vi "PathPlanner_Trajectory25_New.vi"(8 "RobotConfig":T1 {"moduleLocations"."Y" format="%14.3f"; "moduleLocations"."X" format="%14.3f"; "ModuleConfig"."driveMotor"."Jr_KgM2" format="%13.5p"; "ModuleConfig"."driveMotor"."L_H" format="%13.5p"; "ModuleConfig"."driveMotor"."Kt_NMPerAmp" format="%13.5p"; "ModuleConfig"."driveMotor"."KvINV_RadPerSecPerVolt" format="%13.5p"; "ModuleConfig"."driveMotor"."R_Ohms" format="%13.5p"; "ModuleConfig"."driveMotor"."FreeSpeed_RadPerSec" format="%13.5p"; "ModuleConfig"."driveMotor"."FreeCurrent_Amps" format="%13.5p"; "ModuleConfig"."driveMotor"."StallCurrent_Amps" format="%13.5p"; "ModuleConfig"."driveMotor"."StallTorque_NM" format="%13.5p"; "ModuleConfig"."driveMotor"."nominalVoltage_Volts" format="%13.5p"}, 9 "StartingRotation":T5={"VALUE"=0.0, "COS"=1.0, "SIN"=0.0} {"SIN" format="%13.4f"; "COS" format="%13.4f"; "VALUE" format="%13.4f"}, 10 "StartingSpeeds":T10 {"vOmega" format="%10.3f"; "vY" format="%10.3f"; "vX" format="%10.3f"}, 11 "Path":T11={"Reversed"=FALSE, "RotationTargets"=[], "ConstraintZones"=[], "EventMarkers"=[], "GlobalConstraints"={"MaxVelocityMps;"=0.0, "MaxAccelerationMpsSq;"=0.0, "MaxAngularVelRadPsEc;"=0.0, "MaxAngularAccRadPSecSq"=0.0, "Exists"=FALSE, "Unlimited"=FALSE, "NominalVoltageVolts"=12.0}, "GoalEndState"={"VelocityMPS"=0.0, "Rotation"={"VALUE"=0.0, "COS"=1.0, "SIN"=0.0}}, "AllPoints"=[], "Name"="", "Waypoints"=[], "PointTowardsZones"=[], "IdealStartingState"={"VelocityMPS"=0.0, "Rotation"={"VALUE"=1.0, "COS"=0.0, "SIN"=0.0}}, "IsChoreoPath"=FALSE, "PreventFlipping"=FALSE} {"IdealStartingState"."Rotation"."SIN" format="%13.4f"; "IdealStartingState"."Rotation"."COS" format="%13.4f"; "IdealStartingState"."Rotation"."VALUE" format="%13.4f"; "PointTowardsZones"."TargetPosition"."Y" format="%14.3f"; "PointTowardsZones"."TargetPosition"."X" format="%14.3f"; "PointTowardsZones"."RotationOffset"."SIN" format="%13.4f"; "PointTowardsZones"."RotationOffset"."COS" format="%13.4f"; "PointTowardsZones"."RotationOffset"."VALUE" format="%13.4f"; "Waypoints"."nextControl"."Y" format="%14.3f"; "Waypoints"."nextControl"."X" format="%14.3f"; "Waypoints"."anchor"."Y" format="%14.3f"; "Waypoints"."anchor"."X" format="%14.3f"; "Waypoints"."prevControl"."Y" format="%14.3f"; "Waypoints"."prevControl"."X" format="%14.3f"; "AllPoints"."RotationTarget"."rotation"."SIN" format="%13.4f"; "AllPoints"."RotationTarget"."rotation"."COS" format="%13.4f"; "AllPoints"."RotationTarget"."rotation"."VALUE" format="%13.4f"; "AllPoints"."Position"."Y" format="%14.3f"; "AllPoints"."Position"."X" format="%14.3f"; "GoalEndState"."Rotation"."SIN" format="%13.4f"; "GoalEndState"."Rotation"."COS" format="%13.4f"; "GoalEndState"."Rotation"."VALUE" format="%13.4f"; "RotationTargets"."rotation"."SIN" format="%13.4f"; "RotationTargets"."rotation"."COS" format="%13.4f"; "RotationTargets"."rotation"."VALUE" format="%13.4f"}) -> (1 "PathPlannerTrajectoryEvents":T6, 3 "PathPlannerTrajectory":T21 {"States"."ModuleStates"."SWERVE_DRIVE_MODULE_STATE"."Angle"."SIN" format="%13.4f"; "States"."ModuleStates"."SWERVE_DRIVE_MODULE_STATE"."Angle"."COS" format="%13.4f"; "States"."ModuleStates"."SWERVE_DRIVE_MODULE_STATE"."Angle"."VALUE" format="%13.4f"; "States"."ModuleStates"."FieldAngle"."SIN" format="%13.4f"; "States"."ModuleStates"."FieldAngle"."COS" format="%13.4f"; "States"."ModuleStates"."FieldAngle"."VALUE" format="%13.4f"; "States"."ModuleStates"."FieldPos"."Y" format="%14.3f"; "States"."ModuleStates"."FieldPos"."X" format="%14.3f"; "States"."DeltaRot"."SIN" format="%13.4f"; "States"."DeltaRot"."COS" format="%13.4f"; "States"."DeltaRot"."VALUE" format="%13.4f"; "States"."pose"."ROTATION"."SIN" format="%13.4f"; "States"."pose"."ROTATION"."COS" format="%13.4f"; "States"."pose"."ROTATION"."VALUE" format="%13.4f"; "States"."pose"."TRANSLATION"."Y" format="%14.3f"; "States"."pose"."TRANSLATION"."X" format="%14.3f"; "States"."FieldSpeeds"."vOmega" format="%10.3f"; "States"."FieldSpeeds"."vY" format="%10.3f"; "States"."FieldSpeeds"."vX" format="%10.3f"; "States"."Heading"."SIN" format="%13.4f"; "States"."Heading"."COS" format="%13.4f"; "States"."Heading"."VALUE" format="%13.4f"})   [LabVIEW 2019, in "PathPlanner24.lvlib"]
doc: "Generate a PathPlannerTrajectory\n\nInputs: \n - path - cluster - path to generate the trajectory for\n - startingSpeeds - chassis speeds - Starting speeds of the robot when starting the trajectory\n\nOutputs:\n - trajectory - cluster - created trajectory data\n - TrajectoryEvents - cluster - created trajectory events data cluster"
uses:
  PathPlanner24.lvlib
  <vilib>/Rock Robotics/WPI/ThirdParty/JAS_Junk/TrajLib/TypeDef/TRANSLATION2D.ctl
  <vilib>/Rock Robotics/WPI/ThirdParty/JAS_Junk/TrajLib/Trajectory_Library.lvlib
  <vilib>/Rock Robotics/WPI/ThirdParty/JAS_Junk/TrajLib/TypeDef/ROTATION2D.ctl
  TypeDef/PathPlannerPathConstraints.ctl
  ENum/PathPlanner_CommandUtilType_ENUM.ctl
  TypeDef/PathPlannerCommandUtil.ctl
  TypeDef/PathPlannerTrajectoryEvent.ctl
  TypeDef/PathPlannerTrajectoryEvents.ctl
  <vilib>/Rock Robotics/WPI/ThirdParty/JAS_Junk/TrajLib/TypeDef/CHASSIS_SPEEDS.ctl
  <vilib>/Rock Robotics/WPI/ThirdParty/JAS_Junk/TrajLib/TypeDef/POSE2D.ctl
  <vilib>/Rock Robotics/WPI/ThirdParty/JAS_Junk/TrajLib/TypeDef/SWERVE_DRIVE_MODULE_STATE.ctl
  TypeDef/PathPlannerSwerveModTrajState.ctl
  TypeDef/PathPlannerDriveFeedFwds.ctl
  TypeDef/PathPlannerTrajectoryState25.ctl
  TypeDef/PathPlannerTrajectory25.ctl
  TypeDef/PathPlannerRotationTarget.ctl
  TypeDef/PathPlannerConstraintsZone.ctl
  TypeDef/PathPlannerEventMarker.ctl
  TypeDef/PathPlannerGoalEndState.ctl
  TypeDef/PathPlannerPathPoint.ctl
  TypeDef/PathPlannerPath.ctl
  TypeDef/PathPlannerWaypoint.ctl
  TypeDef/PathPlannerPointTowardsZone.ctl
  TypeDef/PathPlannerIdealStartingState.ctl
  <vilib>/Rock Robotics/WPI/ThirdParty/JAS_Junk/TrajLib/TypeDef/DCMOTOR.CTL
  TypeDef/PathPlannerModuleConfig.ctl
  TypeDef/PathPlannerRobotConfig.ctl
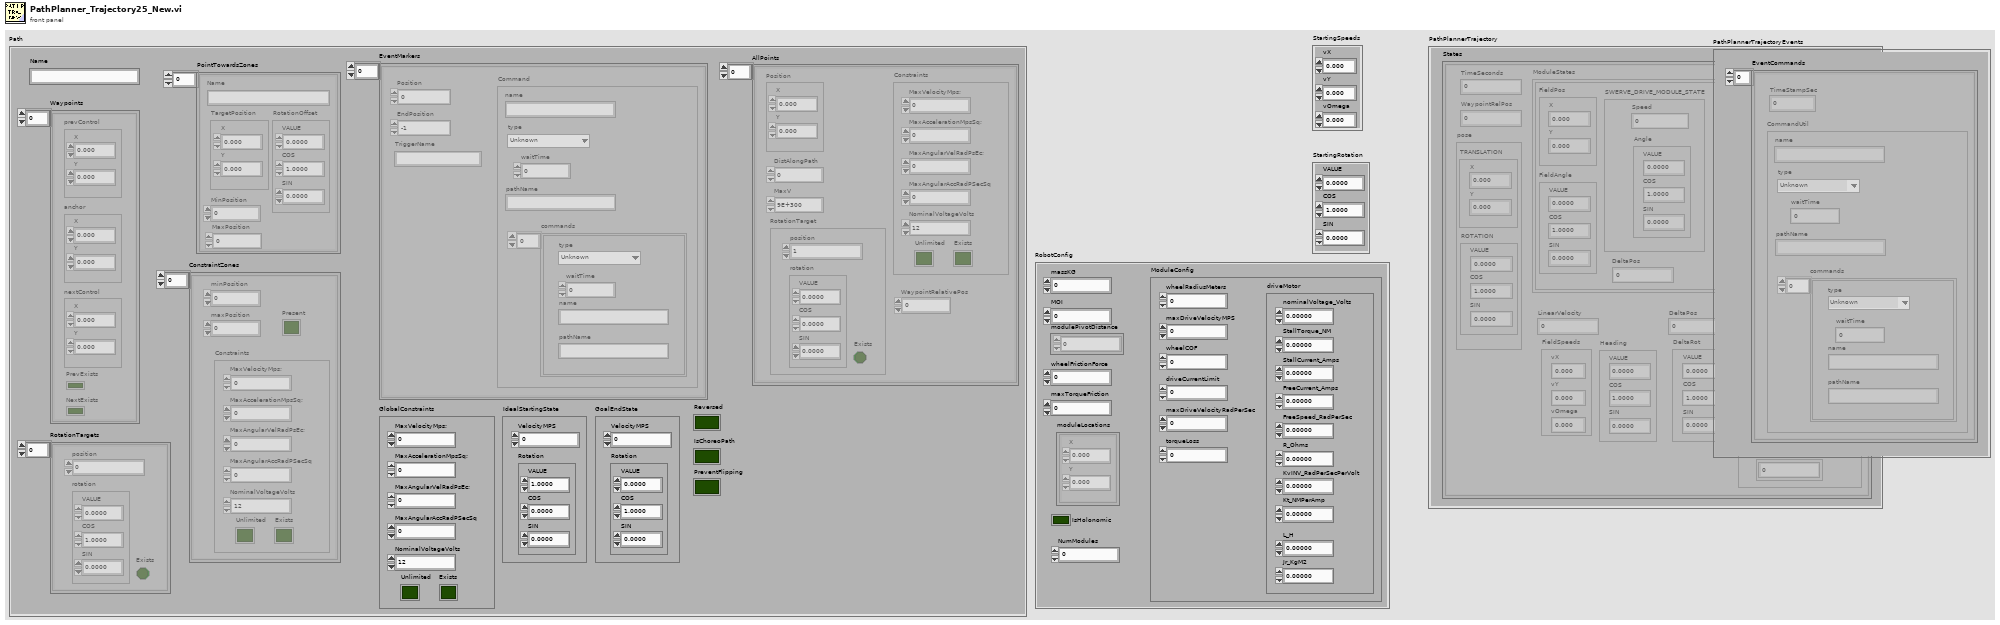
[diagram p1: front panel]
types:
  T1 = typedef "PathPlanner24.lvlib/PathPlannerRobotConfig.ctl" = cluster{"massKG":dbl, "MOI":dbl, "modulePivotDistance":dbl[], "wheelFrictionForce":dbl, "maxTorqueFriction":dbl, "ModuleConfig":T2, "moduleLocations":T4[], "IsHolonomic":bool, "NumModules":i32}
  T2 = typedef "PathPlanner24.lvlib/PathPlannerModuleConfig.ctl" = cluster{"wheelRadiusMeters":dbl, "maxDriveVelocityMPS":dbl, "wheelCOF":dbl, "driveCurrentLimit":dbl, "maxDriveVelocityRadPerSec":dbl, "torqueLoss":dbl, "driveMotor":T3}
  T3 = typedef "Trajectory_Library.lvlib/DCMOTOR.CTL" = cluster{"nominalVoltage_Volts":dbl, "StallTorque_NM":dbl, "StallCurrent_Amps":dbl, "FreeCurrent_Amps":dbl, "FreeSpeed_RadPerSec":dbl, "R_Ohms":dbl, "KvINV_RadPerSecPerVolt":dbl, "Kt_NMPerAmp":dbl, "L_H":dbl, "Jr_KgM2":dbl}
  T4 = typedef "Trajectory_Library.lvlib/TRANSLATION2D.ctl" = cluster{"X":dbl, "Y":dbl}
  T5 = typedef "Trajectory_Library.lvlib/ROTATION2D.ctl" = cluster{"VALUE":dbl, "COS":dbl, "SIN":dbl}
  T6 = typedef "PathPlanner24.lvlib/PathPlannerTrajectoryEvents.ctl" = cluster{"EventCommands":T7[]}
  T7 = typedef "PathPlanner24.lvlib/PathPlannerTrajectoryEvent.ctl" = cluster{"TimeStampSec":dbl, "CommandUtil":T8}
  T8 = typedef "PathPlanner24.lvlib/PathPlannerCommandUtil.ctl" = cluster{"waitTime":dbl, "name":string, "pathName":string, "commands":cluster{"type":T9, "waitTime":dbl, "name":string, "pathName":string}[], "type":T9}
  T9 = typedef "PathPlanner24.lvlib/PathPlanner_CommandUtilType_ENUM.ctl" = enum16{"Unknown", "Wait", "Named", "Path", "Sequential", "Parallel", "Race", "Deadline"}
  T10 = typedef "Trajectory_Library.lvlib/CHASSIS_SPEEDS.ctl" = cluster{"vX":dbl, "vY":dbl, "vOmega":dbl}
  T11 = typedef "PathPlanner24.lvlib/PathPlannerPath.ctl" = cluster{"Reversed":bool, "RotationTargets":T12[], "ConstraintZones":T13[], "EventMarkers":T15[], "GlobalConstraints":T14, "GoalEndState":T16, "AllPoints":T17[], "Name":string, "Waypoints":T18[], "PointTowardsZones":T19[], "IdealStartingState":T20, "IsChoreoPath":bool, "PreventFlipping":bool}
  T12 = typedef "PathPlanner24.lvlib/PathPlannerRotationTarget.ctl" = cluster{"position":dbl, "rotation":T5, "Exists":bool}
  T13 = typedef "PathPlanner24.lvlib/PathPlannerConstraintsZone.ctl" = cluster{"minPosition":dbl, "maxPosition":dbl, "Constraints":T14, "Present":bool}
  T14 = typedef "PathPlanner24.lvlib/PathPlannerPathConstraints.ctl" = cluster{"MaxVelocityMps;":dbl, "MaxAccelerationMpsSq;":dbl, "MaxAngularVelRadPsEc;":dbl, "MaxAngularAccRadPSecSq":dbl, "Exists":bool, "Unlimited":bool, "NominalVoltageVolts":dbl}
  T15 = typedef "PathPlanner24.lvlib/PathPlannerEventMarker.ctl" = cluster{"Position":dbl, "Command":T8, "TriggerName":string, "EndPosition":dbl}
  T16 = typedef "PathPlanner24.lvlib/PathPlannerGoalEndState.ctl" = cluster{"VelocityMPS":dbl, "Rotation":T5}
  T17 = typedef "PathPlanner24.lvlib/PathPlannerPathPoint.ctl" = cluster{"Position":T4, "DistAlongPath":dbl, "MaxV":dbl, "Constraints":T14, "RotationTarget":T12, "WaypointRelativePos":dbl}
  T18 = typedef "PathPlanner24.lvlib/PathPlannerWaypoint.ctl" = cluster{"prevControl":T4, "anchor":T4, "nextControl":T4, "PrevExists":bool, "NextExists":bool}
  T19 = typedef "PathPlanner24.lvlib/PathPlannerPointTowardsZone.ctl" = cluster{"RotationOffset":T5, "Name":string, "TargetPosition":T4, "MinPosition":dbl, "MaxPosition":dbl}
  T20 = typedef "PathPlanner24.lvlib/PathPlannerIdealStartingState.ctl" = cluster{"VelocityMPS":dbl, "Rotation":T5}
  T21 = typedef "PathPlanner24.lvlib/PathPlannerTrajectory25.ctl" = cluster{"States":T22[]}
  T22 = typedef "PathPlanner24.lvlib/PathPlannerTrajectoryState25.ctl" = cluster{"TimeSeconds":dbl, "LinearVelocity":dbl, "Heading":T5, "Constraints":T14, "DeltaPos":dbl, "FieldSpeeds":T10, "pose":T23, "DeltaRot":T5, "ModuleStates":T24[], "WaypointRelPos":dbl, "Feedforwards":T26}
  T23 = typedef "Trajectory_Library.lvlib/POSE2D.ctl" = cluster{"TRANSLATION":T4, "ROTATION":T5}
  T24 = typedef "PathPlanner24.lvlib/PathPlannerSwerveModTrajState.ctl" = cluster{"FieldPos":T4, "FieldAngle":T5, "DeltaPos":dbl, "SWERVE_DRIVE_MODULE_STATE":T25}
  T25 = typedef "Trajectory_Library.lvlib/SWERVE_DRIVE_MODULE_STATE.ctl" = cluster{"Speed":dbl, "Angle":T5}
  T26 = typedef "PathPlanner24.lvlib/PathPlannerDriveFeedFwds.ctl" = cluster{"accelerationsMPSSq":dbl[], "linearForcesNewtons":dbl[], "torqueCurrentsAmps":dbl[], "robotRelativeForcesXNewtons":dbl[], "robotRelativeForcesYNewtons":dbl[]}
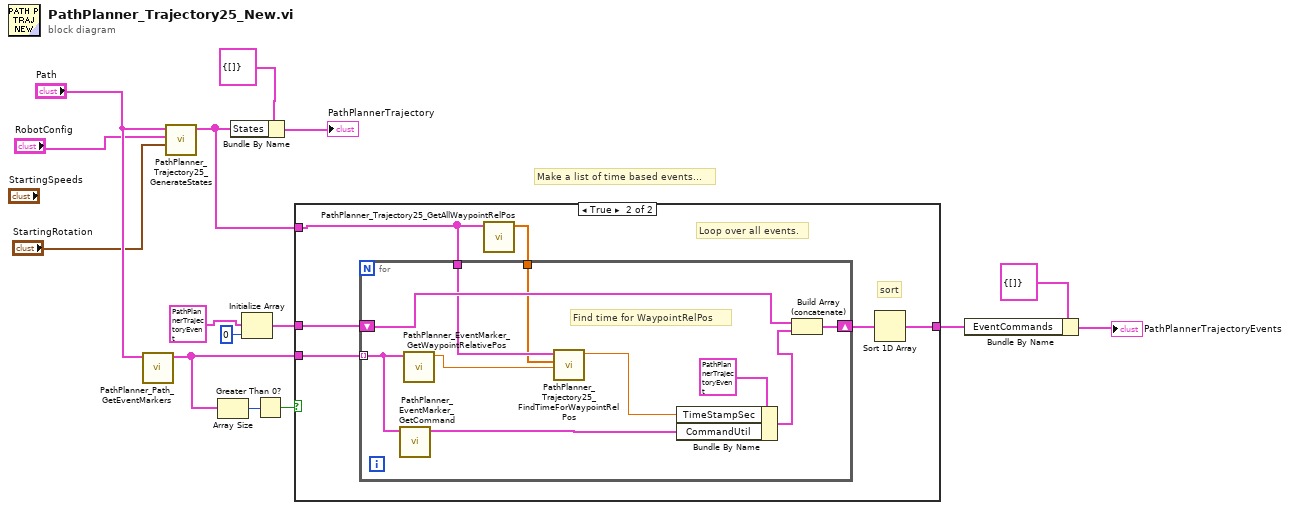
[diagram p0: block diagram]
diagram:
  # "Make a list of time based events..."
  n1 = call "PathPlanner_Path_GetEventMarkers.vi"("PathPlannerPath"="Path") -> ("EventMarkers"=w10:T15[])  [unwired: 10 in]
  n2 = call "PathPlanner_Trajectory25_GenerateStates.vi"("StartingRotation"="StartingRotation", "RobotConfig"="RobotConfig", "PathPlannerPath"="Path") -> ("PathPlannerStates"=w9:T22[])  [unwired: 8 in]
  n3 = Array Size(array=w10) -> (size(s)=w12:i32)
  n4 = Bundle By Name(cluster=T21 {"States"=[]} ("PathPlannerState25"), "States"=w9) -> (→"PathPlannerTrajectory":T21)
  n5 = Initialize Array(T7 {"TimeStampSec"=0.0, "CommandUtil"={"waitTime"=0.0, "name"="", "pathName"="", "commands"=[], "type"=enum."Unknown"}} ("TrajectoryEvent"), 0 ("dimension size")) -> (w6:T7[])
  n6 = Greater Than 0?(x=w12) -> (x > 0?=w11:bool)
  n7 = case shown="True" w11 {
    tunnel: [w16 w19] -> w3
    tunnel: w10 -> [_ w22]
    tunnel: w9 -> [_ w18]
    tunnel: w6 -> [w16 w21]
    frame False {
    }
    frame True {
      # "Loop over all events."
      # "sort"
      n8 = call "PathPlanner_Trajectory25_GetAllWaypointRelPos.vi"("PathPlannerStates"=w18) -> ("AllWaypointRelPos"=w17:dbl[])  [unwired: 10 in]
      n9 = for {
        shift-right: [w27] -> w20
        shift-left: w21 -> [w31]
        tunnel: w22 -> [w32] mode=indexing
        tunnel: w18 -> [w26]
        tunnel: w17 -> [w25]
        # "Find time for WaypointRelPos"
        n10 = call "PathPlanner_EventMarker_GetCommand.vi"("in EventMarker"=w32) -> ("Command"=w29:T8)  [unwired: 10 in]
        n11 = call "PathPlanner_EventMarker_GetWaypointRelativePos.vi"("in EventMarker"=w32) -> ("WaypointRelativePos"=w24:dbl)  [unwired: 10 in]
        n12 = call "PathPlanner_Trajectory25_FindTimeForWaypointRelPos.vi"("WaypointRelPos"=w24, "AllWayPointRelPos"=w25, "PathPlannerStates"=w26) -> ("Time_Secs"=w23:dbl)  [unwired: 8 in]
        n13 = Bundle By Name(cluster=T7 {"TimeStampSec"=0.0, "CommandUtil"={"waitTime"=0.0, "name"="", "pathName"="", "commands"=[], "type"=enum."Unknown"}} ("TrajectoryEvent"), "TimeStampSec"=w23, "CommandUtil"=w29) -> (w28:T7)
        n14 = Build Array (concatenate)(w31, w28) -> (w27:T7[])
      }
      n15 = Sort 1D Array(array=w20) -> (sorted array=w19:T7[])
    }
  }
  n16 = Bundle By Name(cluster=T6 {"EventCommands"=[]} ("PathPlannerTrajectoryEvents"), "EventCommands"=w3) -> (→"PathPlannerTrajectoryEvents":T6)
